vi "Default.vi"(9 "balls":T7[](array[typedef]), 10 "Robot in":T1, 11 "IA State":T6={"our_robots"=[], "enemy_robots"=[], "balls"=[], "geometry"={"field_length"=0, "field_width"=0, "goal_width"=0, "goal_depth"=0, "center_circle_radius"=0, "defense_width"=0, "defense_depth"=0, "free_kick_from_defense_dist"=0, "penalty_spot_from_field_line_dist"=0, "penalty_line_from_spot_dist"=0, "half_moon_depth"=0, "half_moon_width"=0}, "IA Judge"={"stage"="", "command"="", "our_goalie_id"=0.0, "enemy_goalie_id"=0.0, "command enum"=enum."Halt", "Time"=enum."Azul"}, "Received Timestamp"=timestamp(0 s since 1904-01-01), "Events"={"Touch"=FALSE, "id touch"=0.0, "Ball out of \nVision"=FALSE, "Ball inside \nGoalie area"=FALSE, "Robot not responding"=FALSE, "Robots responding status"=[1.0, 1.0, 1.0, 1.0, 1.0, 1.0], "Enemy Ball \nPossession"=FALSE, "Id ini Possession"=0.0, "Ball Possesion"=FALSE, "Id Possesion"=0.0, "Ball at\nour goal side"=FALSE, "Ball at\ntouchline"=FALSE, "Ball at\nenemy goal side"=FALSE}}) -> (3 "Cluster de saída":T1)   [LabVIEW 2018]
doc: "Função que lida com o atacante quando em \"Default\"."
uses:
  Path Planning/RRT/PathDest.ctl
  Intel/Functions Enum.ctl
  Intel/AttackerStates.ctl
  Path Planning/RRT/PathDests.ctl
  Core/AI Robot.ctl
  Core/AI Ball.ctl
  Core/Field Size.ctl
  Intel/Command Enum.ctl
  Core/AI Judge.ctl
  Util/Events/Events.ctl
  Core/AI Input.ctl
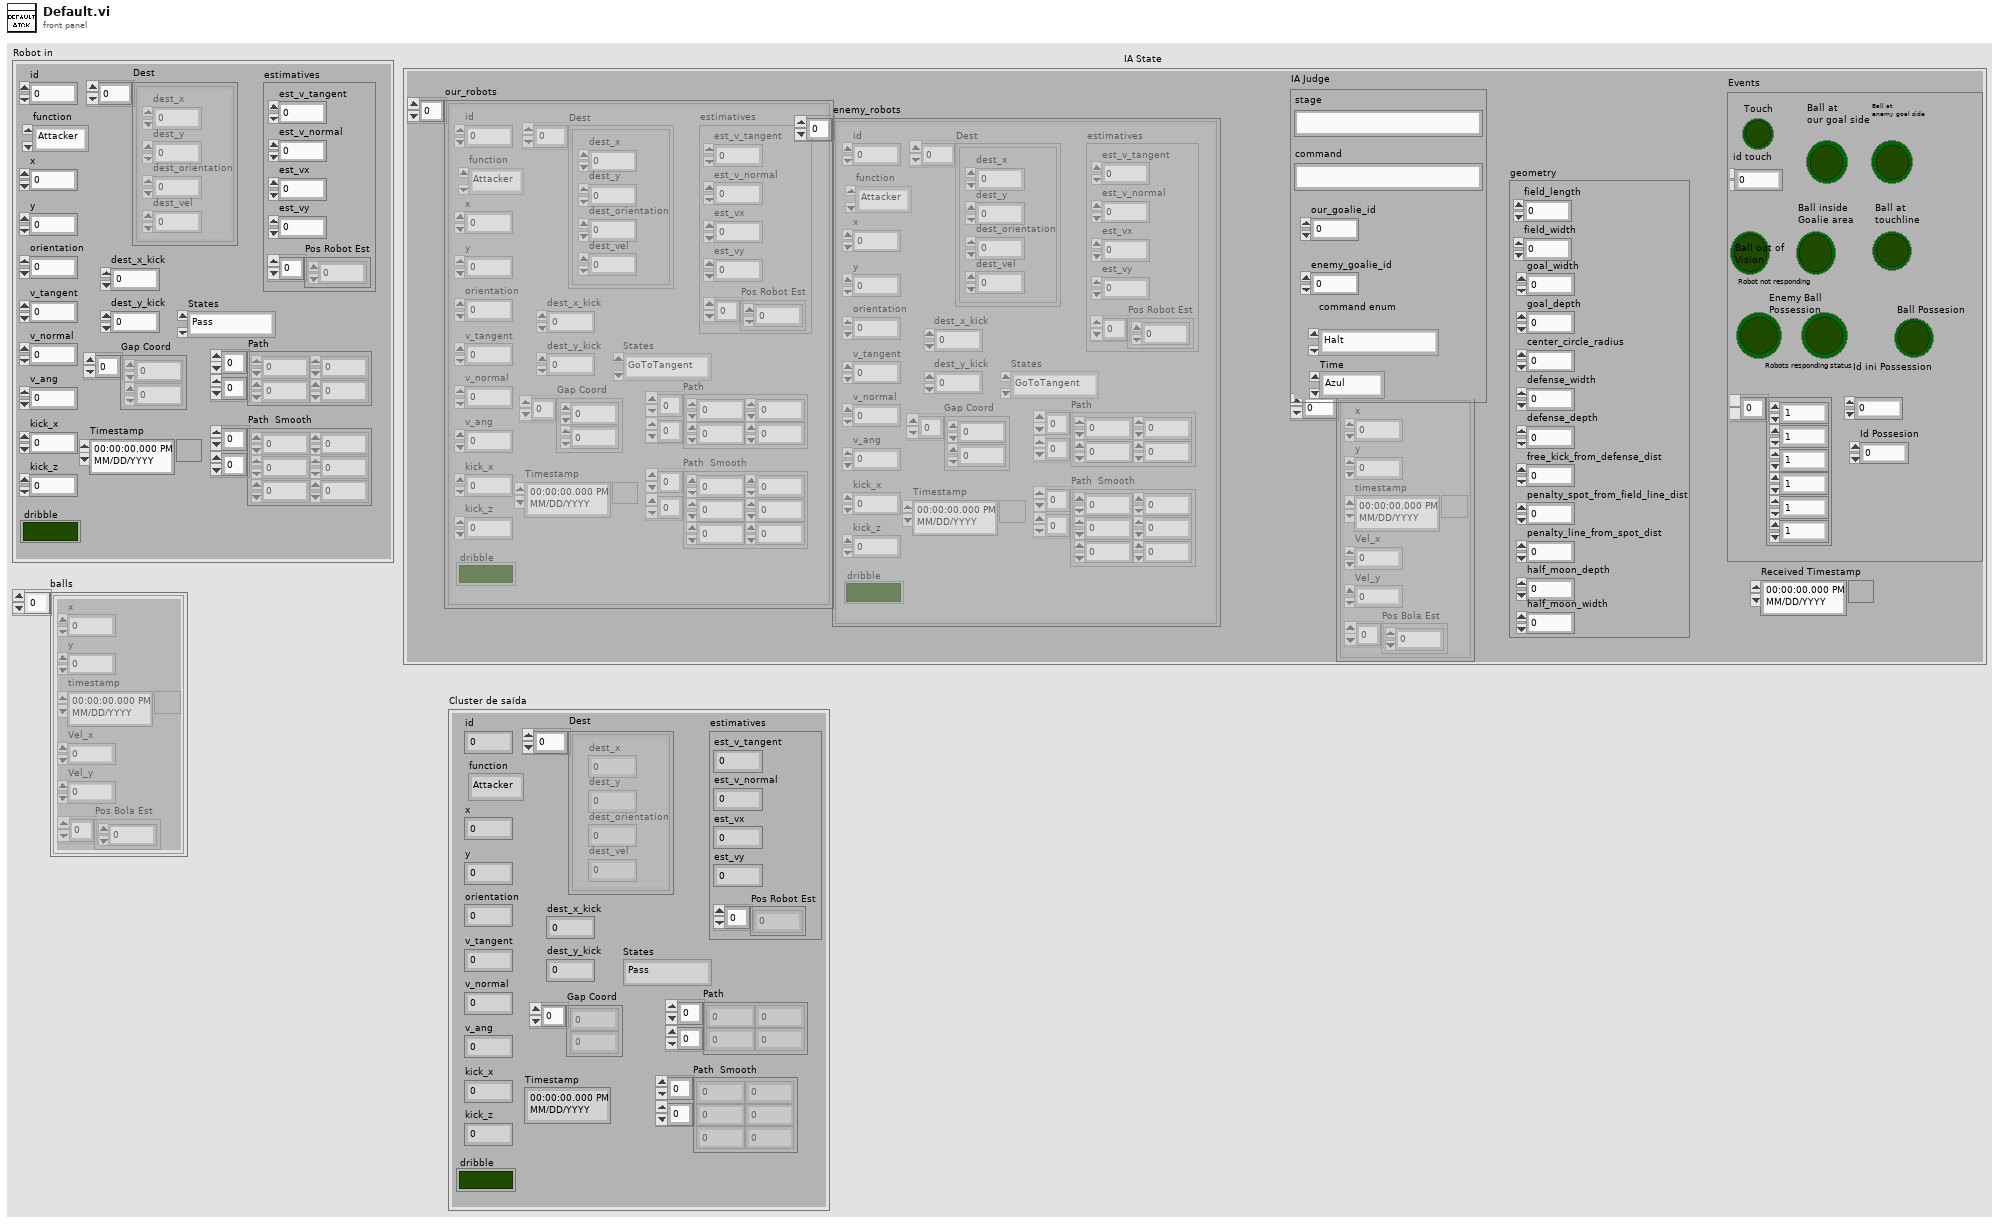
[diagram p1: front panel]
types:
  T1 = typedef "AI Robot.ctl" = cluster{"id":u32, "function":T2, "x":dbl, "y":dbl, "orientation":dbl, "v_tangent":dbl, "v_normal":dbl, "v_ang":dbl, "kick_x":dbl, "kick_z":dbl, "dribble":bool, "Timestamp":timestamp, "estimatives":cluster{"est_v_tangent":dbl, "est_v_normal":dbl, "est_vx":dbl, "est_vy":dbl, "Pos Robot Est":dbl[]}, "dest_x_kick":dbl, "dest_y_kick":dbl, "Gap Coord":dbl[], "States":T3, "Path ":dbl[][], "Path  Smooth":dbl[][], "Dest":T4}
  T2 = typedef "Functions Enum.ctl" = enum16{"Attacker", "Goalie", "Defender", "Striker", "Goto 0", "Dummy", "Kicker", "ZigZag"}
  T3 = typedef "AttackerStates.ctl" = enum16{"Pass", "GoToTangent", "BallGetting", "GoToKick", "Rotate anti-clockwise", "Rotate Clockwise", ""}
  T4 = typedef "PathDests.ctl" = T5[]
  T5 = typedef "PathDest.ctl" = cluster{"dest_x":dbl, "dest_y":dbl, "dest_orientation":dbl, "dest_vel":dbl}
  T6 = typedef "AI Input.ctl" = cluster{"our_robots":T1[], "enemy_robots":T1[], "balls":T7[], "geometry":T8, "IA Judge":T9, "Received Timestamp":timestamp, "Events":T11}
  T7 = typedef "AI Ball.ctl" = cluster{"x":dbl, "y":dbl, "timestamp":timestamp, "Vel_x":dbl, "Vel_y":dbl, "Pos Bola Est":dbl[]}
  T8 = typedef "Field Size.ctl" = cluster{"field_length":u32, "field_width":u32, "goal_width":u32, "goal_depth":u32, "center_circle_radius":u32, "defense_width":u32, "defense_depth":u32, "free_kick_from_defense_dist":u32, "penalty_spot_from_field_line_dist":u32, "penalty_line_from_spot_dist":u32, "half_moon_depth":u32, "half_moon_width":u32}
  T9 = typedef "AI Judge.ctl" = cluster{"stage":string, "command":string, "our_goalie_id":dbl, "enemy_goalie_id":dbl, "command enum":T10, "Time":enum16{"Azul", "Amarelo"}}
  T10 = typedef "Command Enum.ctl" = enum16{"Halt", "Stop", "Force Start", "PKA Normal Start", "Prepare Kickoff Ally", "PKE Normal Start", "Prepare Kickoff Enemy", "Prepare Penalty Ally", "PPA Normal Start", "Prepare Penalty Enemy", "PPE Normal Start", "Ball Placement Enemy Up", "Ball Placement Enemy Down", "Ball Placement Ally Up", "Ball Placement Ally Mid", "Ball Placement Ally Down", "Indirect Free Enemy", "Indirect Free Ally", "Timeout Enemy", "Timeout Ally", "Goal Enemy", "Goal Ally", "Normal Half Time", "Extra Time Break", "Extra Half Time", "None", "Post Game"}
  T11 = typedef "Events.ctl" = cluster{"Touch":bool, "id touch":dbl, "Ball out of \nVision":bool, "Ball inside \nGoalie area":bool, "Robot not responding":bool, "Robots responding status":dbl[], "Enemy Ball \nPossession":bool, "Id ini Possession":dbl, "Ball Possesion":bool, "Id Possesion":dbl, "Ball at\nour goal side":bool, "Ball at\ntouchline":bool, "Ball at\nenemy goal side":bool}
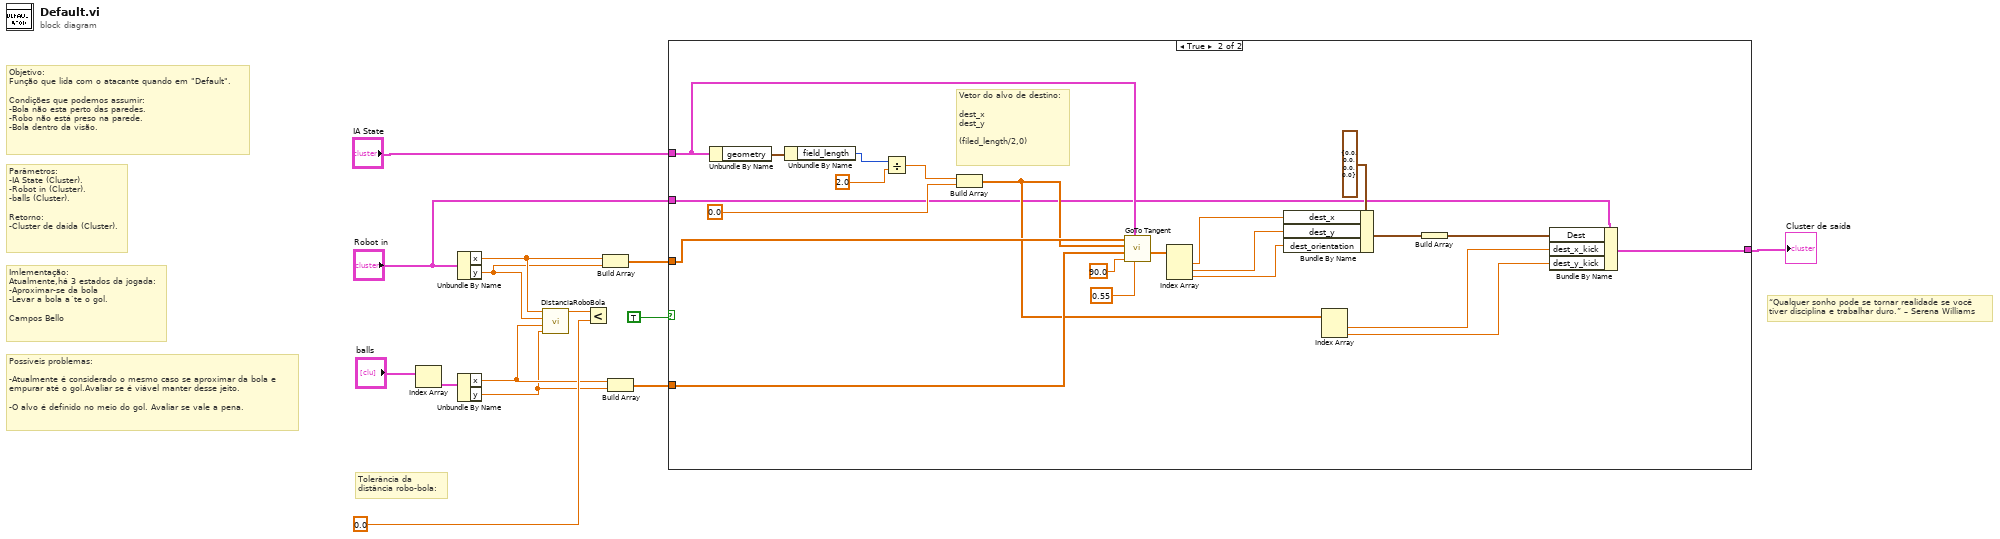
[diagram p0: block diagram]
diagram:
  # "“Qualquer sonho pode se tornar realidade se você \ntiver disciplina e trabalhar duro.” – Serena Williams"
  # "Possíveis problemas:\n\n-Atualmente é considerado o mesmo caso se aproximar da bola e\nempurar até o gol.Avaliar se é viável manter desse jeito.\n\n-O alvo é definido no meio do gol. Avaliar se vale a pena."
  # "Imlementação:\nAtualmente,há 3 estados da jogada:\n-Aproximar-se da bola\n-Levar a bola a´te o gol.\n\nCampos Bello"
  # "Parâmetros:\n-IA State (Cluster).\n-Robot in (Cluster).\n-balls (Cluster).\n\nRetorno:\n-Cluster de daída (Cluster)."
  # "Objetivo:\nFunção que lida com o atacante quando em \"Default\".\n\nCondições que podemos assumir:\n-Bola não esta perto das paredes.\n-Robo não está preso na parede.\n-Bola dentro da visão."
  # "Tolerância da\ndistância robo-bola:"
  n1 = Index Array(array="balls") -> (element=w13:T7)  [unwired: 1 in]
  n2 = Unbundle By Name("Robot in") -> ("x"=w10:dbl, "y"=w9:dbl)
  n3 = Unbundle By Name(w13) -> ("x"=w7:dbl, "y"=w6:dbl)
  n4 = call "DistanciaRoboBola.vi"("Y bola"=w6, "X bola"=w7, "Y robo"=w9, "X robo"=w10) -> ("Distância"=w11:dbl)  [unwired: 5 in, 2 out]
  n5 = Less?(x=w11, y=0.0) -> ()  [unwired: 1 out]
  n6 = Build Array(w10, w9) -> (w8:dbl[])
  n7 = Build Array(w7, w6) -> (w5:dbl[])
  n8 = case shown="True" TRUE {
    tunnel: w8 -> [_ w29]
    tunnel: w5 -> [_ w28]
    tunnel: "IA State" -> [_ w27]
    tunnel: "Robot in" -> [_ w16]
    tunnel: [_ w15] -> w1
    frame False {
    }
    frame True {
      # "Vetor do alvo de destino:\n\ndest_x\ndest_y\n\n(filed_length/2,0)"
      n9 = Unbundle By Name(w27) -> ("geometry"=w34:T8)
      n10 = Unbundle By Name(w34) -> ("field_length"=w33:u32)
      n11 = Divide(x=w33, y=2.0) -> (x/y=w31:dbl)
      n12 = Build Array(w31, 0.0) -> (w17:dbl[])
      n13 = call "GoTo Tangent.vi"("Cone de chute"=0.55, "IA State Input in"=w27, "distance between ball and robot"=90.0, "Ball"=w28, "Target"=w17, "R"=w29) -> ("Destination"=w21:dbl[])  [unwired: 4 in, 1 out]
      n14 = Index Array(array=w21) -> (element #1=w20:dbl, element #2=w19:dbl, element #3=w18:dbl)  [unwired: 3 in]
      n15 = Bundle By Name(cluster=T5 {"dest_x"=0.0, "dest_y"=0.0, "dest_orientation"=0.0, "dest_vel"=0.0} ("element"), "dest_x"=w20, "dest_y"=w19, "dest_orientation"=w18) -> (w25:T5)
      n16 = Index Array(array=w17) -> (element #1=w23:dbl, element #2=w22:dbl)  [unwired: 2 in]
      n17 = Build Array(w25) -> (w24:T5[])
      n18 = Bundle By Name(cluster=w16, "Dest"=w24, "dest_x_kick"=w23, "dest_y_kick"=w22) -> (w15:T1)
    }
  }
  "Cluster de saída" <- w1
